vi "PID Calculus Motor 2.vi"(3 "Current":u16, 4 "PID Controls Motor 1":T1={"PID gains"={"proportional gain (Kc)"=1.0, "integral gain (Kc*Ts/Ti)"=1.66796875, "derivative gain (Kc*Td/Ts)"=0.0}, "reset?"=FALSE, "Velocity wanted (Counts/Interval)"=0, "Velocity Interval (uSec)"=0, "Actual Velocity (Counts/Interval)"=0.0} {"Actual Velocity (Counts/Interval)" format="%.2f"}) -> (0 "PID Output Motor 2":i16, 1 "Direction Motor 2":bool, 2 "PID Pulse Lenght Motor 2":i16)   [LabVIEW 2013]
uses:
  <vilib>/addons/control/pid/pid.llb/PID (DBL).vi
  <vilib>/addons/control/pid/NI_PID_pid.lvlib
panel:
  out "Velocity Interval (uSec)":i32
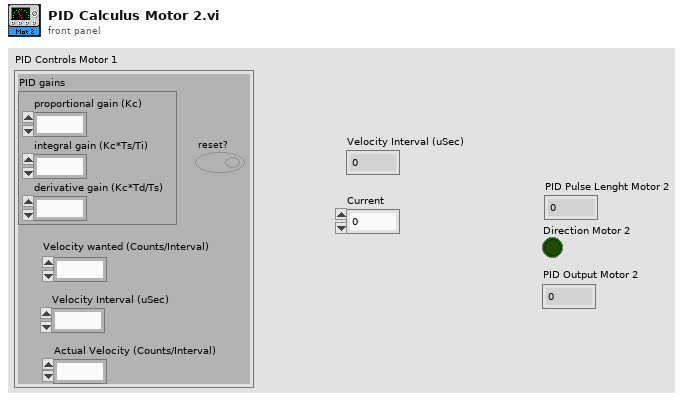
[diagram p1: front panel]
types:
  T1 = cluster{"PID gains":cluster{"proportional gain (Kc)":fxp<+/-,16,8>, "integral gain (Kc*Ts/Ti)":fxp<+/-,16,8>, "derivative gain (Kc*Td/Ts)":fxp<+/-,16,8>}, "reset?":bool, "Velocity wanted (Counts/Interval)":i16, "Velocity Interval (uSec)":i32, "Actual Velocity (Counts/Interval)":dbl}
  T2 = cluster{"proportional gain (Kc)":fxp<+/-,16,8>, "integral gain (Kc*Ts/Ti)":fxp<+/-,16,8>, "derivative gain (Kc*Td/Ts)":fxp<+/-,16,8>}
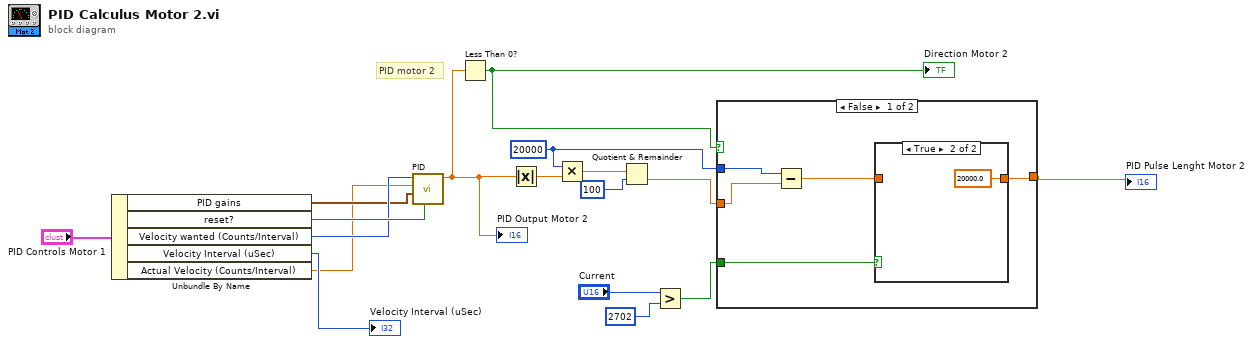
[diagram p0: block diagram]
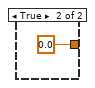
[diagram p4: hidden frame]
diagram:
  w3 = i16 20000 ("x")
  # "PID motor 2"
  n1 = Unbundle By Name("PID Controls Motor 1") -> ("PID gains"=w9:T2, "reset?"=w11:bool, "Velocity wanted (Counts/Interval)"=w10:i16, "Velocity Interval (uSec)"=→"Velocity Interval (uSec)":i32, "Actual Velocity (Counts/Interval)"=w8:dbl)
  n2 = call-poly <vilib>:"PID.vi"("reinitialize? (F)"=w11, "PID gains"=w9, "process variable"=w8, "setpoint"=w10) -> ("output"=w15:dbl)  [unwired: 6 in, 1 out]
  "PID Output Motor 2" <- w15
  n3 = Less Than 0?(x=w15) -> (x < 0?=w4:bool)
  "Direction Motor 2" <- w4
  n4 = Absolute Value(x=w15) -> (abs(x)=w13:dbl)
  n5 = Multiply(x=w3, y=w13) -> (x*y=w14:dbl)
  n6 = Quotient & Remainder(x=w14, y=i16 100) -> (floor(x/y)=w2:dbl)  [unwired: 1 out]
  n7 = Greater?(x="Current", y=u16 2702) -> (0:w5:bool)
  n8 = case shown="False" w4 {
    tunnel: w2 -> [w21 w25]
    tunnel: w3 -> [w22 _]
    tunnel: [w18 w26] -> w1
    tunnel: w5 -> [w20 w27]
    frame False {
      n9 = Subtract(x=w22, y=w21) -> (x-y=w19:dbl)
      n10 = case shown="True" w20 {
        tunnel: w19 -> [w23 _]
        tunnel: [w23 20000.0] -> w18
        frame False {
        }
        frame True {
        }
      }
    }
    frame True {
      n11 = case shown="False" w27 {
        tunnel: [w28 0.0] -> w26
        tunnel: w25 -> [w28 _]
        frame False {
        }
        frame True {
        }
      }
    }
  }
  "PID Pulse Lenght Motor 2" <- w1
